vi "flicker test with zero3.vi"() -> ()   [LabVIEW 2011]
uses:
  <instrlib>/Tektronix DPO MSO 2000 4000 Series/Public/Data/Data_Low Level/Fetch Waveform (Waveform Data Type).vi
  <instrlib>/Tektronix DPO MSO 2000 4000 Series/Tektronix DPO MSO 2000 4000 Series.lvlib
panel:
  in  "Channel (0: Channel 1)":u16(ring) items=["Channel 1", "Channel 2", "Channel 3", "Channel 4", "Math", "Reference 1", "Reference 2", "Reference 3", "Reference 4", "D0", "D1", "D2", "D3", "D4", "D5", "D6", "D7", "D8", "D9", "D10", "D11", "D12", "D13", "D14", "D15", "Amplitude", "Frequency", "Phase", "Normal", "Average", "Maximum Peak Hold", "Minimum Peak Hold"]
  in  "Maximum Time (10000ms)":u32=10000
  in  "VISA Resource Name":refnum<visa-resource-name>
  out "Filename Out":path
  out "appended path":path
  out "data":waveform(dbl)(graph)
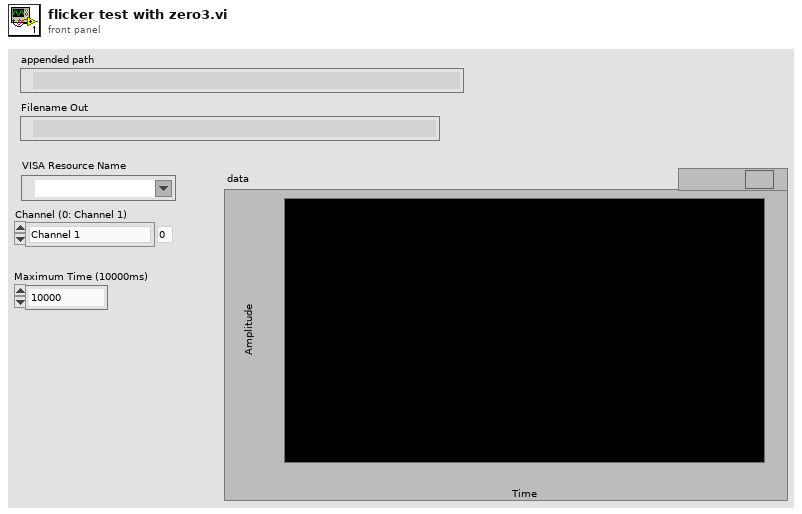
[diagram p1: front panel]
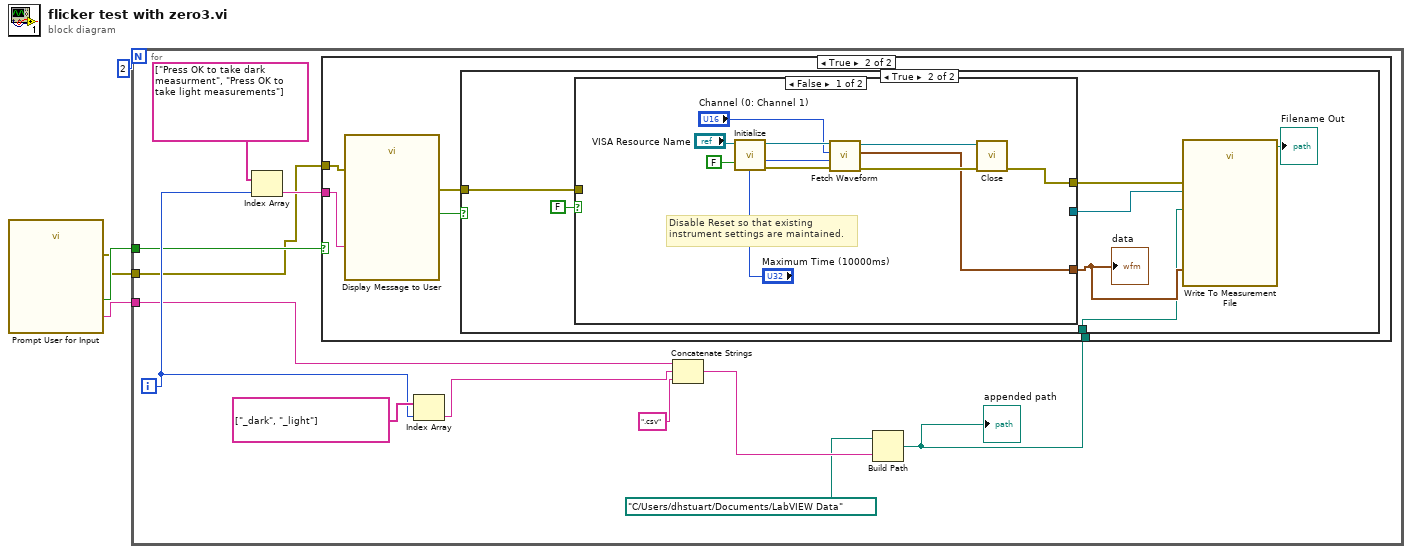
[diagram p0: block diagram]
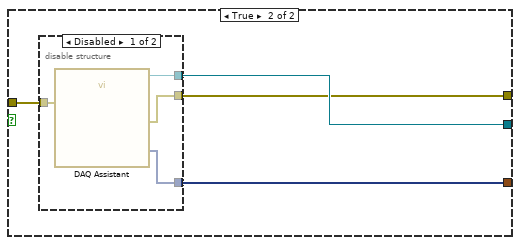
[diagram p4: hidden frame]
diagram:
  n1 = call "Prompt User for Input"() -> ("file_name"=w3:string, "OK"=w2:bool, "error out"=w1:errorcluster)  [unwired: 17 in]
  n2 = for {
    N: 2 -> [_]
    tunnel: w3 -> [w7]
    tunnel: w2 -> [w6]
    tunnel: w1 -> [w5]
    i -> [w11]
    n3 = Index Array(array=string[] ["Press OK to take dark measurment", "Press OK to take light measurements"], index=w11) -> (element=w15:string)
    n4 = Index Array(array=string[] ["_dark", "_light"], index=w11) -> (element=w9:string)
    n5 = Concatenate Strings(w7, w9, ".csv" ("string")) -> (w14:string)
    n6 = Build Path(base path=path "C:/Users/dhstuart/Documents/LabVIEW Data", name or relative path=w14) -> (appended path=w13:path)
    "appended path" <- w13
    n7 = case shown="True" w6 {
      tunnel: w15 -> [_ w19]
      tunnel: w13 -> [_ w18]
      tunnel: w5 -> [_ w17]
      frame False {
      }
      frame True {
        n8 = call "Display Message to User"("error in (no error)"=w17, "Message"=w19) -> ("error out"=w21:errorcluster, "OK"=w20:bool)  [unwired: 8 in]
        n9 = case shown="True" w20 {
          tunnel: w21 -> [_ w28]
          tunnel: w18 -> [_ w24]
          frame False {
          }
          frame True {
            n10 = case shown="False" FALSE {
              tunnel: w28 -> [_ w42]
              tunnel: [_ w41] -> w27
              tunnel: [w30 w40] -> w26
              tunnel: [w29 w39] -> w25
              frame False {
                # "Disable Reset so that existing\ninstrument settings are maintained."
                n11 = call <instrlib>:"Initialize.vi"("Reset (True)"=FALSE ("Reset? (T: Yes)"), "VISA resource name"="VISA Resource Name") -> ("error out"=w35:errorcluster, "VISA resource name out"=w36:refnum<visa-resource-name>)  [unwired: 8 in]
                n12 = call-poly <instrlib>:"Fetch Waveform.vi"("error in (no error)"=w35, "Maximum Time (10000ms)"="Maximum Time (10000ms)", "Channel (0: Channel 1)"="Channel (0: Channel 1)", "VISA resource name"=w36) -> ("error out"=w34:errorcluster, "Waveform Data"=w30:waveform(dbl), "VISA resource name out"=w31:refnum<visa-resource-name>)  [unwired: 5 in]
                n13 = call <instrlib>:"Close.vi"("error in (no error)"=w34, "VISA resource name"=w31) -> ("error out"=w29:errorcluster)  [unwired: 9 in]
              }
              frame True {
                n14 = disable-structure shown="Disabled" {
                  disable-tunnel: w42 -> [w46 _]
                  disable-tunnel: [w45 _] -> w41
                  disable-tunnel: [w44 _] -> w40
                  disable-tunnel: [w43 _] -> w39
                  frame Disabled {
                    n15 = call "DAQ Assistant"("error in"=w46) -> ("task out"=w45:refnum<k21>, "data"=w44:dynamicdata, "error out"=w43:errorcluster)  [unwired: 16 in]
                  }
                  frame Enabled {
                  }
                }
              }
            }
            "data" <- w26
            n16 = call "Write To Measurement File"("Signals"=w26, "error in (no error)"=w25, "Filename"=w24, "DAQmx Task"=w27) -> ("Filename Out"=→"Filename Out":path)  [unwired: 13 in, 2 out]
          }
        }
      }
    }
  }
